vi "DQMH-GenNet Create Message Queue.vi"(8 "error in (no error)":errorcluster) -> (0 "error out":errorcluster, 3 "Message Queue out":refnum<class "DQMH-GenNet Message Queue.lvclass">)   [LabVIEW 2020, in "hse-gennet.lvlib" / "DQMH-GenNet Message Queue.lvclass"]
doc: "This is the modified \"Create Message Queue\" VI for DQMH Generic Networking\n\n____\nHAMPEL SOFTWARE ENGINEERING v3.8.0 (2023-12-18 14:41)"
uses:
  DQMH-GenNet Message Queue.lvclass
  DQMH-GenNet Message Queue.lvclass/DQMH-GenNet Message Queue.ctl
  <vilib>/Delacor/Delacor QMH/Libraries/Message Queue_class/Delacor_lib_QMH_Message Queue.lvclass
  <vilib>/Delacor/Delacor QMH/Libraries/Message Queue_class/Delacor_lib_QMH_Enqueue Message (Single).vi
  <vilib>/Delacor/Delacor QMH/Libraries/Message Queue_class/Delacor_lib_QMH_Message--cluster.ctl
  C:/Program Files (x86)/National Instruments/LabVIEW 2020/vi.lib/Delacor/Delacor QMH/Libraries/Message Queue_class/Delacor_lib_QMH_Message Queue.lvclass
  C:/LabVIEW/hse-application-template/TEMPLATE_Source/Libraries/hse-libraries/Source/hse-gennet/DQMH-GenNet Message Queue.lvclass
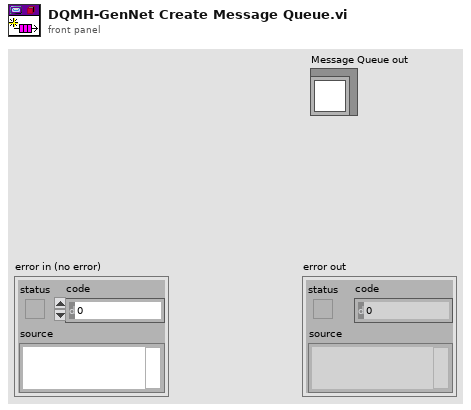
[diagram p1: front panel]
types:
  T1 = typedef "Delacor_lib_QMH_Message Queue.lvclass/Delacor_lib_QMH_Message--cluster.ctl" = cluster{"Message":string, "Message Data":variant}
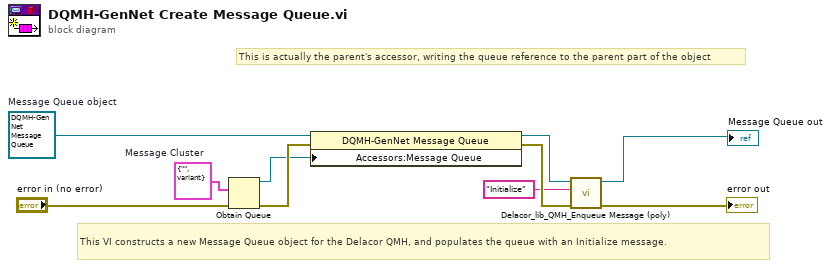
[diagram p0: block diagram]
diagram:
  w6 = T1 {"Message"="", "Message Data"=variant}  # Message Cluster
  w9 = refnum<class "DQMH-GenNet Message Queue.lvclass"> refnum  # Message Queue object
  # "This is actually the parent's accessor, writing the queue reference to the parent part of the object"
  # "This VI constructs a new Message Queue object for the Delacor QMH, and populates the queue with an Initialize message."
  n1 = Obtain Queue(element data type=w6, error in (no error)="error in (no error)") -> (queue out=w1:refnum<queue>, error out=w4:errorcluster)  [unwired: 3 in, 1 out]
  n2 = property class="DQMH-GenNet Message Queue"(reference=w9, error in=w4, "Accessors:Message Queue"=w1) -> (reference out=w7:refnum<class "DQMH-GenNet Message Queue.lvclass">, error out=w3:errorcluster)
  n3 = call-poly <vilib>:"Delacor_lib_QMH_Enqueue Message (poly).vi"("error in"=w3, "Message"="Initialize", "Message Queue in"=w7) -> ("error out"=→"error out":errorcluster, "Message Queue out"=→"Message Queue out":refnum<class "DQMH-GenNet Message Queue.lvclass">)  [unwired: 7 in]
